vi "Wait.vi"(8 "error in (no error)":errorcluster, 10 "Time(ms)":i32=200) -> (0 "error out":errorcluster)   [LabVIEW 2016]
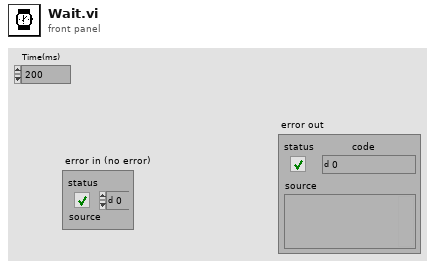
[diagram p1: front panel]
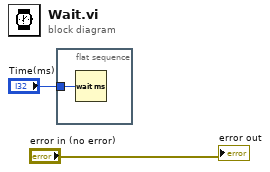
[diagram p0: block diagram]
diagram:
  n1 = flat-sequence {
    tunnel: "Time(ms)" -> [w3]
    frame #0 {
      n2 = Wait (ms)(milliseconds to wait=w3) -> ()  [unwired: 1 out]
    }
  }
  "error out" <- "error in (no error)"
